vi "F Dwf Analog Out Frequency Info.vi"(7 "phzMax":dbl, 8 "error in (no error)":errorcluster, 9 "phzMin":dbl, 10 "idxChannel":i32, 11 "hdwf":i32) -> (0 "error out":errorcluster, 1 "phzMin out":dbl, 3 "function return":i32, 5 "phzMax out":dbl)   [LabVIEW 2019, in "Olasdwf.lvlib"]
doc: "DWFAPI int FDwfAnalogOutFrequencyInfo(HDWF hdwf, int idxChannel, double *phzMin, double *phzMax);"
uses:
  Olasdwf.lvlib
  Windows/System32/dwf.dll
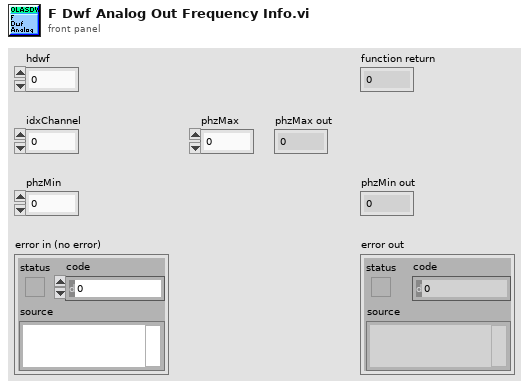
[diagram p1: front panel]
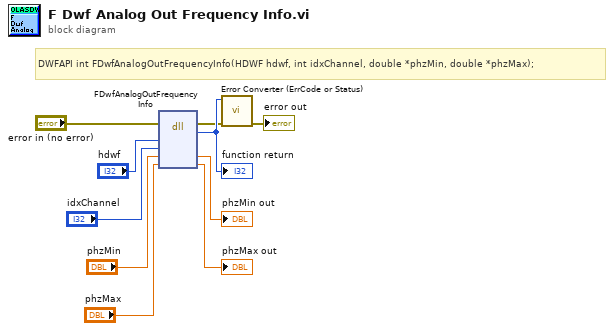
[diagram p0: block diagram]
diagram:
  # "DWFAPI int FDwfAnalogOutFrequencyInfo(HDWF hdwf, int idxChannel, double *phzMin, double *phzMax);"
  n1 = dll-call lib="C:/Windows/System32/dwf.*" fn="FDwfAnalogOutFrequencyInfo"(error in="error in (no error)", "hdwf"="hdwf", "idxChannel"="idxChannel", "phzMin"="phzMin", "phzMax"="phzMax") -> (error out=w2:errorcluster, w10:i32, "phzMin"=→"phzMin out":dbl, "phzMax"=→"phzMax out":dbl)  [unwired: 4 in, 1 out]
  "function return" <- w10
  n2 = call "Error Converter (ErrCode or Status).vi"("error in (no error)"=w2, "error code"=w10) -> ("error out"=→"error out":errorcluster)  [unwired: 9 in]
